vi "SubSystems.vi"(8 "error in":errorcluster) -> ()   [LabVIEW 2020]
doc: "This VI calls the various robot subsystems that will then run in parallel. New subSystems will automatlically script code to make the call."
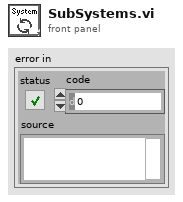
[diagram p1: front panel]
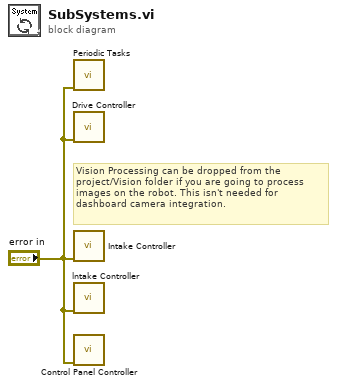
[diagram p0: block diagram]
diagram:
  # "Vision Processing can be dropped from the\nproject/Vision folder if you are going to process\nimages on the robot. This isn't needed for\ndashboard camera integration."
  n1 = call "Periodic Tasks.vi"("error in"="error in") -> ()  [unwired: 1 in, 10 out]
  n2 = call "Drive Controller.vi"("error in"="error in") -> ()  [unwired: 11 in]
  n3 = call "Intake Controller.vi"("error in"="error in") -> ()  [unwired: 11 in]
  n4 = call "lntake Controller.vi"("error in"="error in") -> ()  [unwired: 11 in]
  n5 = call "Control Panel Controller.vi"("error in"="error in") -> ()  [unwired: 11 in]
